vi "Keyence.Cmd.Version.vi"(8 "error in (no error)":errorcluster, 9 "Timeout [ms] (1000)":i32=1000, 11 "connection ID":refnum<k5>) -> (0 "error out":errorcluster, 1 "version":string, 2 "model":string, 3 "connection ID out":refnum<k5>, 4 "cmd ok":bool)   [LabVIEW 2016]
panel:
  out "response":string
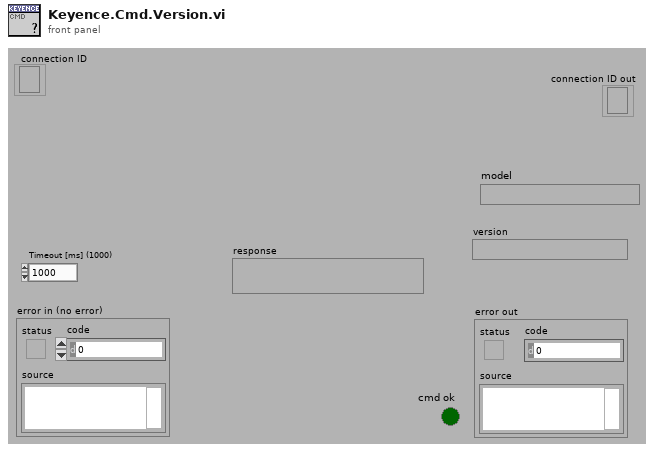
[diagram p1: front panel]
types:
  T1 = enum16{"Standard", "Buffered", "CRLF", "Immediate"}
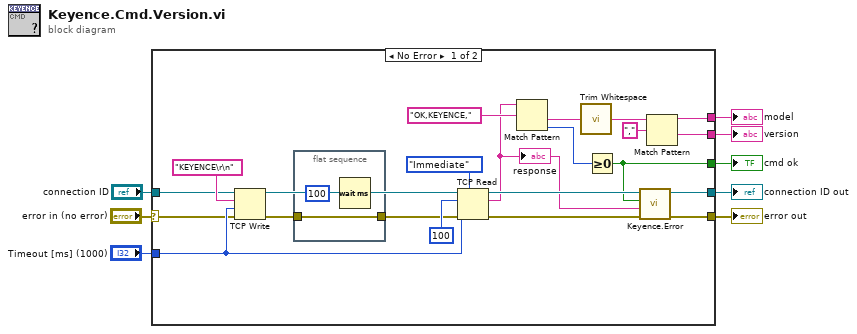
[diagram p0: block diagram]
diagram:
  n1 = case shown="No Error" "error in (no error)" {
    selector: "error in (no error)" -> [w14 w33]
    tunnel: [w12 w33] -> w8
    tunnel: "Timeout [ms] (1000)" -> [w29 _]
    tunnel: [w16 _] -> w5
    tunnel: [w10 _] -> w4
    tunnel: [w17 _] -> w3
    tunnel: "connection ID" -> [w15 w32]
    tunnel: [w13 w32] -> w1
    frame No Error {
      n2 = TCP Write(connection ID=w15, data in="KEYENCE\r\n" ("concatenated string"), error in (no error)=w14, 9:w29) -> (connection ID out=w28:refnum<k5>, error out=w25:errorcluster)  [unwired: 1 out]
      n3 = flat-sequence {
        tunnel: w25 -> [w31]
        tunnel: [w31] -> w24
        frame #0 {
          n4 = Wait (ms)(milliseconds to wait=u32 100) -> ()  [unwired: 1 out]
        }
      }
      n5 = TCP Read(connection ID=w28, bytes to read=100, error in (no error)=w24, 7:T1."Immediate" ("mode (standard)"), 9:w29) -> (connection ID out=w13:refnum<k5>, data out=w9:string, error out=w11:errorcluster)
      "response" <- w9
      n6 = Match Pattern(string=w9, regular expression="OK,KEYENCE,") -> (after substring=w20:string, offset past match=w21:i32)  [unwired: 1 in, 2 out]
      n7 = call <vilib>:"Trim Whitespace.vi"("string"=w20) -> ("trimmed string"=w19:string)  [unwired: 1 in]
      n8 = Greater Or Equal To 0?(x=w21) -> (x >= 0?=w10:bool)
      n9 = call "Keyence.Error.vi"("error in (no error)"=w11, "Response"=w9, "Cmd ok"=w10) -> ("error out"=w12:errorcluster)  [unwired: 8 in]
      n10 = Match Pattern(string=w19, regular expression=",") -> (before substring=w17:string, after substring=w16:string)  [unwired: 1 in, 2 out]
    }
    frame Error {
    }
  }
  "error out" <- w8
  "version" <- w5
  "cmd ok" <- w4
  "model" <- w3
  "connection ID out" <- w1
